vi "Simulate Synchronous Controller.vi"(0 "Cal Climber in":T11, 3 "Execution Mode":T13, 4 "Wheel Speed (mm/s)":i16(slide)=100 scale=0.0..500.0, 5 "error in (no error)":errorcluster, 6 "C DLL path":path=path "D:/Users/jjensen/workspace/Simulated iRobot Navigation/Release/libSimulated iRobot Navigation.dll", 7 "Play Button":bool, 8 "accel smoothing (0-1)":dbl=0.1, 9 "Stop Simulation":bool) -> (11 "Diagram Display":picture, 13 "iRobot Sensors (graphical)":T12 {"Right Wheel (mm/s)" scale=-500.0..500.0; "Left Wheel (mm/s)" scale=-500.0..500.0}, 14 "Cal Climber out":T11, 15 "Statechart Inputs":T1={"net distance (mm)"=0, "net angle (deg)"=0, "Max Wheel Speed (mm/s)"=0, "accelerometer"={"x axis (g)"=0.0, "y axis (g)"=0.0, "z axis (g)"=0.0}, "iRobot Sensors"={"Bumps + Wheel Drops"={"Wheeldrop Caster"=FALSE, "Wheeldrop Left"=FALSE, "Wheeldrop Right"=FALSE, "Bump Left"=FALSE, "Bump Right"=FALSE}, "Wall"=FALSE, "Cliff Left"=FALSE, "Cliff Front Left"=FALSE, "Cliff Front Right"=FALSE, "Cliff Right"=FALSE, "Virtual Wall"=FALSE, "Low-Side Driver + Wheel Overcurrent"={"Low-Side Driver 0"=FALSE, "Low-Side Driver 1"=FALSE, "Low-Side Driver 2"=FALSE, "Left Wheel"=FALSE, "Right Wheel"=FALSE}, "Infrared"=255, "Buttons"={"Advance"=FALSE, "Play"=FALSE}, "Distance (mm)"=0, "Angle (deg)"=0, "Charging State"=enum."Not Charging", "Voltage (mV)"=0, "Current (mA)"=0, "Battery Temperature (deg C)"=0, "Battery Charge (mAh)"=0, "Battery Capacity (mAh)"=0, "Wall Signal (0-4095)"=0, "Cliff Left Signal (0-4095)"=0, "Cliff Front Left Signal (0-4095)"=0, "Cliff Front Right Signal (0-4095)"=0, "Cliff Right Signal (0-4095)"=0, "Cargo Bay Digital Inputs"={"Digital Input 0"=FALSE, "Digital Input 1"=FALSE, "Digital Input 2"=FALSE, "Digital Input 3"=FALSE, "Device Detect"=FALSE}, "Cargo Bay Analog Signal (0-1023)"=0, "Charging Sources Available"={"Internal Charger"=FALSE, "Home Base"=FALSE}, "OI Mode"=enum."Off", "Song Number"=0, "Song Playing"=FALSE, "Number of Stream Packets"=0, "Requested Velocity (mm/s)"=0, "Requested Radius (mm)"=0, "Requested Right Wheel Velocity (mm/s)"=0, "Requested Left Wheel Velocity (mm/s)"=0}, "Is Simulator?"=FALSE} {"iRobot Sensors"."Infrared" format="%02x"; "accelerometer"."z axis (g)" format="%.3f"; "accelerometer"."y axis (g)" format="%.3f"; "accelerometer"."x axis (g)" format="%.3f"; "Max Wheel Speed (mm/s)" scale=0.0..500.0}, 17 "Active States":string[](array[string]), 19 "error out":errorcluster)   [LabVIEW 2013]
uses:
  iRobot Sensors.ctl
  Simulate Execution Mode.ctl
  Simulate iRobot.ctl
  <instrlib>/DC Motor Controller/HAIOL/DC Motor Controller.lvclass
  iRobot Navigation State Machine.lvsc/Inputs.ctl
  Accelerometer.ctl
  iRobot/Sensor/Sensor Group 6.ctl
  iRobot/Sensor/Bumps + Wheel Drops.ctl
  iRobot/Sensor/Low-Side Driver + Wheel Overcurrent.ctl
  iRobot/Sensor/Buttons.ctl
  iRobot/Sensor/Charging State.ctl
  iRobot/Sensor/Cargo Bay Digital Inputs.ctl
  iRobot/Sensor/Charging Sources Available.ctl
  iRobot/Sensor/OI Mode.ctl
  iRobot Navigation State Machine.lvsc
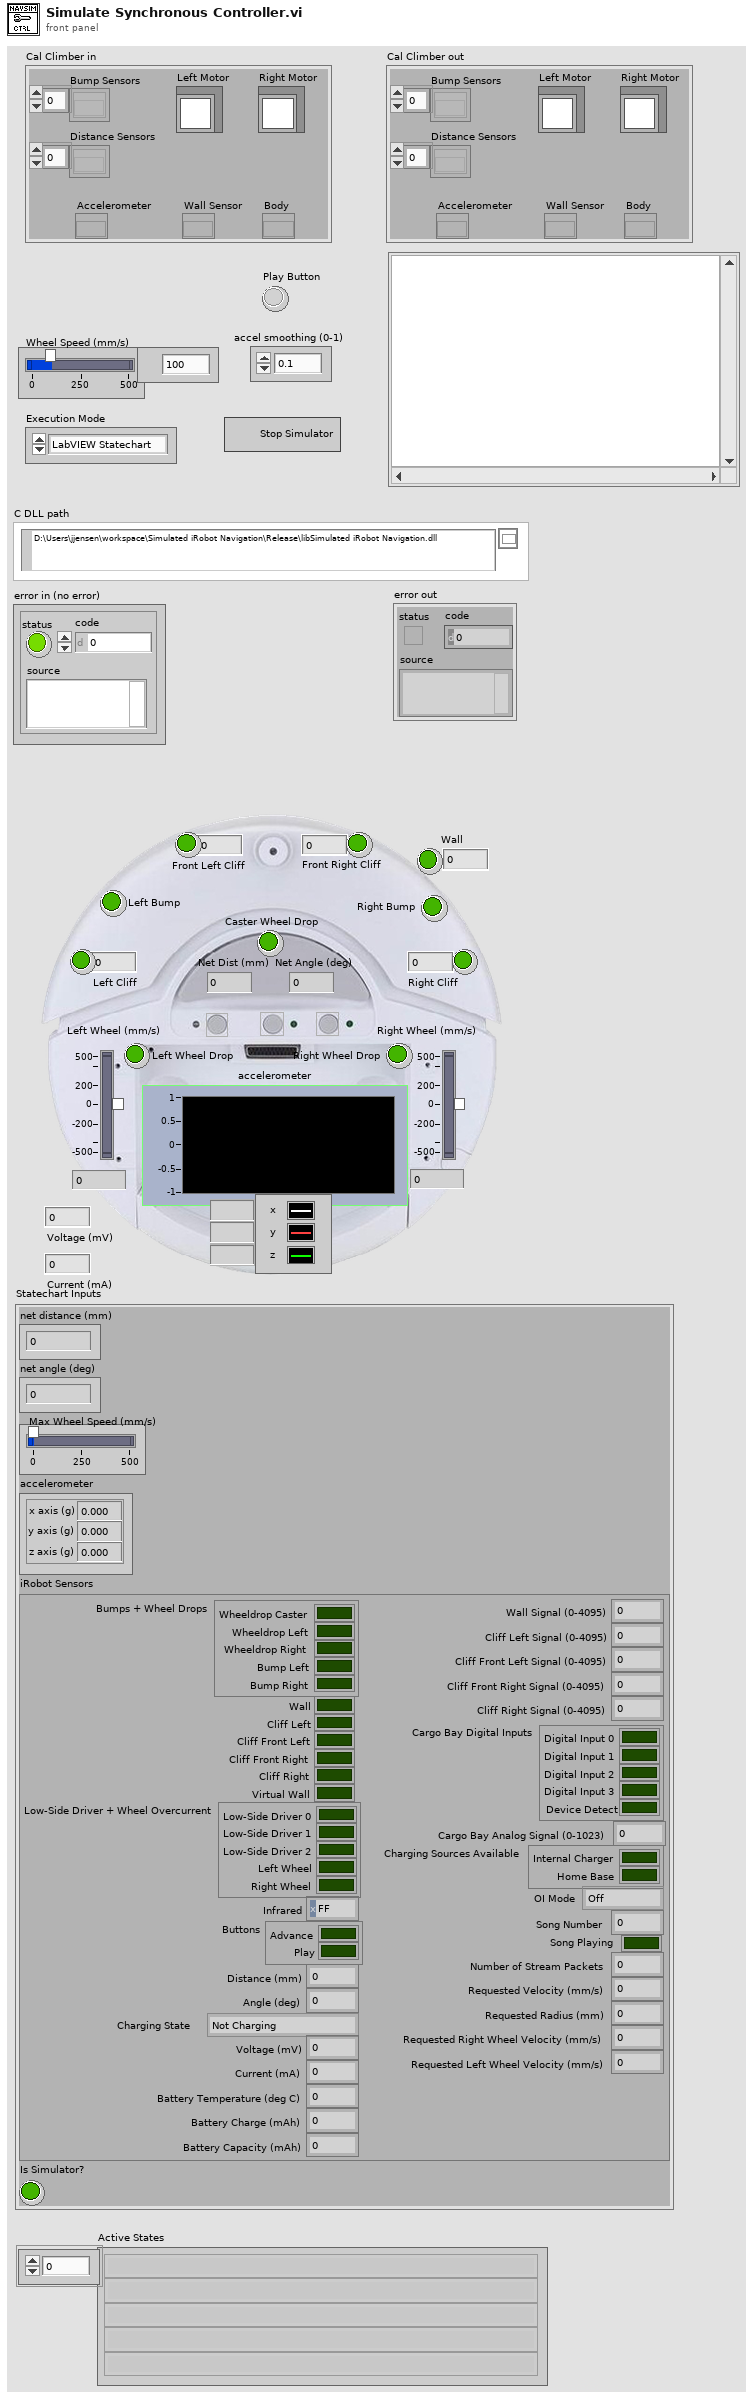
[diagram p1: front panel]
types:
  T1 = typedef "iRobot Navigation State Machine.lvsc/Inputs.ctl" = cluster{"net distance (mm)":i32, "net angle (deg)":i32, "Max Wheel Speed (mm/s)":i16, "accelerometer":T2, "iRobot Sensors":T3, "Is Simulator?":bool}
  T2 = typedef "Accelerometer.ctl" = cluster{"x axis (g)":dbl, "y axis (g)":dbl, "z axis (g)":dbl}
  T3 = typedef "Sensor Group 6.ctl" = cluster{"Bumps + Wheel Drops":T4, "Wall":bool, "Cliff Left":bool, "Cliff Front Left":bool, "Cliff Front Right":bool, "Cliff Right":bool, "Virtual Wall":bool, "Low-Side Driver + Wheel Overcurrent":T5, "Infrared":u8, "Buttons":T6, "Distance (mm)":i32, "Angle (deg)":i32, "Charging State":T7, "Voltage (mV)":u16, "Current (mA)":i16, "Battery Temperature (deg C)":i8, "Battery Charge (mAh)":u16, "Battery Capacity (mAh)":u16, "Wall Signal (0-4095)":u16, "Cliff Left Signal (0-4095)":u16, "Cliff Front Left Signal (0-4095)":u16, "Cliff Front Right Signal (0-4095)":u16, "Cliff Right Signal (0-4095)":u16, "Cargo Bay Digital Inputs":T8, "Cargo Bay Analog Signal (0-1023)":u16, "Charging Sources Available":T9, "OI Mode":T10, "Song Number":u8, "Song Playing":bool, "Number of Stream Packets":u8, "Requested Velocity (mm/s)":i16, "Requested Radius (mm)":i16, "Requested Right Wheel Velocity (mm/s)":i16, "Requested Left Wheel Velocity (mm/s)":i16}
  T4 = typedef "Bumps + Wheel Drops.ctl" = cluster{"Wheeldrop Caster":bool, "Wheeldrop Left":bool, "Wheeldrop Right":bool, "Bump Left":bool, "Bump Right":bool}
  T5 = typedef "Low-Side Driver + Wheel Overcurrent.ctl" = cluster{"Low-Side Driver 0":bool, "Low-Side Driver 1":bool, "Low-Side Driver 2":bool, "Left Wheel":bool, "Right Wheel":bool}
  T6 = typedef "Buttons.ctl" = cluster{"Advance":bool, "Play":bool}
  T7 = typedef "Charging State.ctl" = enum16{"Not Charging", "Reconditioning Charging", "Full Charging", "Trickle Charging", "Waiting", "Charging Fault Condition"}
  T8 = typedef "Cargo Bay Digital Inputs.ctl" = cluster{"Digital Input 0":bool, "Digital Input 1":bool, "Digital Input 2":bool, "Digital Input 3":bool, "Device Detect":bool}
  T9 = typedef "Charging Sources Available.ctl" = cluster{"Internal Charger":bool, "Home Base":bool}
  T10 = typedef "OI Mode.ctl" = enum16{"Off", "Passive", "Safe", "Full"}
  T11 = typedef "Simulate iRobot.ctl" = cluster{"Bump Sensors":refnum<k20>[], "Distance Sensors":refnum<k20>[], "Accelerometer":refnum<k20>, "Wall Sensor":refnum<k20>, "Body":refnum<k20>, "Left Motor":refnum<class "DC Motor Controller.lvclass">, "Right Motor":refnum<class "DC Motor Controller.lvclass">}
  T12 = typedef "iRobot Sensors.ctl" = cluster{"Caster Wheel Drop":bool, "Left Wheel Drop":bool, "Right Wheel Drop":bool, "Left Bump":bool, "Right Bump":bool, "Left Cliff":bool, "Front Left Cliff":bool, "Front Right Cliff":bool, "Right Cliff":bool, "Wall":bool, "Net Dist (mm)":i32, "Net Angle (deg)":i32, "Wall":u16, "Left Cliff":u16, "Front Left Cliff":u16, "Front Right Cliff":u16, "Right Cliff":u16, "Left Wheel (mm/s)":i16, "Right Wheel (mm/s)":i16, "accelerometer":T2, "Voltage (mV)":dbl, "Current (mA)":dbl}
  T13 = typedef "Simulate Execution Mode.ctl" = enum16{"LabVIEW Statechart", "C Statechart"}
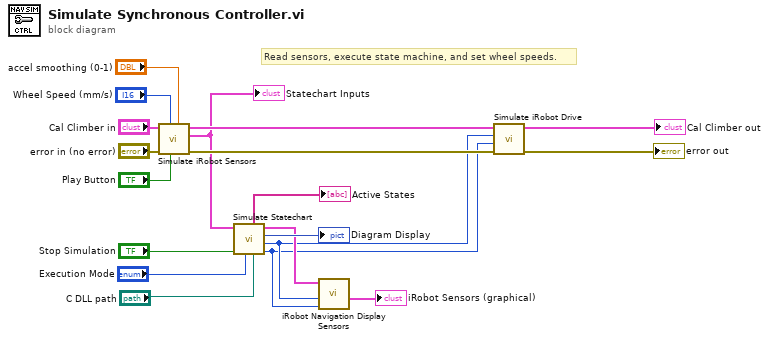
[diagram p0: block diagram]
diagram:
  # "Read sensors, execute state machine, and set wheel speeds."
  n1 = call "Simulate iRobot Sensors.vi"("accel smoothing (0-1)"="accel smoothing (0-1)", "Play Button"="Play Button", "Wheel Speed (mm/s)"="Wheel Speed (mm/s)", "error in"="error in (no error)", "Cal Climber"="Cal Climber in") -> ("error out"=w12:errorcluster, "Statechart Inputs"=w5:T1, "Cal Climber"=w11:T11)  [unwired: 4 in]
  "Statechart Inputs" <- w5
  n2 = call "Simulate Statechart.vi"("C DLL path"="C DLL path", "Execution Mode"="Execution Mode", "stop"="Stop Simulation", "Statechart Inputs In"=w5) -> ("Left Wheel Speed (mm/s)"=w1:i16, "Right Wheel Speed (mm/s)"=w2:i16, "Diagram Display"=→"Diagram Display":picture, "Statechart Inputs Out"=w6:T1, "Active States"=→"Active States":string[])  [unwired: 3 in]
  n3 = call "iRobot Navigation Display Sensors.vi"("Left Wheel (mm/s)"=w1, "Right Wheel (mm/s)"=w2, "Statechart Inputs"=w6) -> ("iRobot Sensors (graphical)"=→"iRobot Sensors (graphical)":T12)  [unwired: 6 in]
  n4 = call "Simulate iRobot Drive.vi"("error in"=w12, "Left Wheel Speed (mm/s)"=w1, "Right Wheel Speed (mm/s)"=w2, "Cal Climber"=w11) -> ("error out"=→"error out":errorcluster, "Cal Climber"=→"Cal Climber out":T11)  [unwired: 6 in]
